vi "Core Actor - Init User Events.vi"(8 "error in (no error)":errorcluster, 11 "Parent_Class in":refnum<class "Message_Distributor_Class.lvclass">) -> (0 "error out":errorcluster, 3 "Parent_Class out":refnum<class "Message_Distributor_Class.lvclass">)   [LabVIEW 2023, in "Actor_Message_Distributor.lvlib" / "Message_Distributor_Class.lvclass"]
uses:
  Message_Distributor_Class.lvclass
  Usr Ev/Distributor - Ctrl - Action.ctl
  Message_Distributor_Class.lvclass/Message_Distributor_Class.ctl
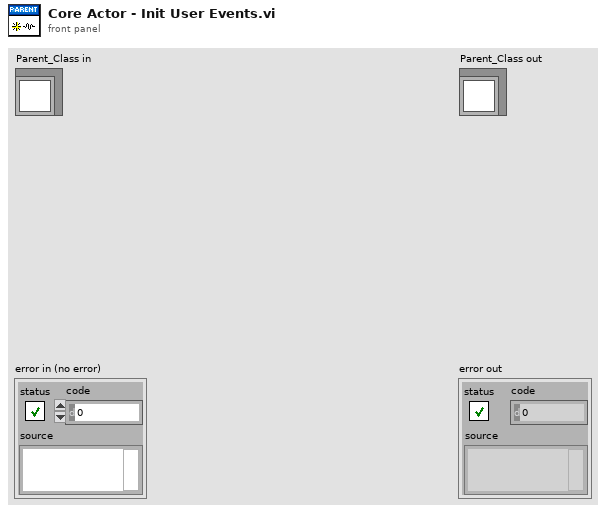
[diagram p1: front panel]
types:
  T1 = typedef "Actor_Message_Distributor.lvlib/Message_Distributor_Class.lvclass/Distributor - Ctrl - Action.ctl" = enum16{"Reg Ev", "Get Refs", "Close Ev", "Populate Enum with Events"}
  T2 = typedef "Actor_Message_Distributor.lvlib/Message_Distributor_Class.lvclass/Distributor - Ctrl - Usr Ev Ref.ctl" = cluster{"SEND MESSAGE Ev":cluster{"Data":refnum<user-event>}, "STOP_ACTOR Ev":cluster{"Data":refnum<user-event>}, "INIT_ACTOR Ev":cluster{"Data":refnum<user-event>}, "START Ev":cluster{"Data":refnum<user-event>}, "STOP Ev":cluster{"Data":refnum<user-event>}, "GET Ev":cluster{"Data":refnum<user-event>}, "SET Ev":cluster{"Data":refnum<user-event>}, "ERROR_HANDLER Ev":cluster{"Data":refnum<user-event>}, "RESET Ev":cluster{"Data":refnum<user-event>}, "DISPATCH MESSAGE 2 CHILDS Ev":cluster{"Data":refnum<user-event>}, "ECU RESET Ev":cluster{"Data":refnum<user-event>}, "T4 Ev":cluster{"Data":refnum<user-event>}}
  T3 = typedef "Actor_Message_Distributor.lvlib/Message_Distributor_Class.lvclass/Distributor - Ctrl - Usr Ev Reg - Refs.ctl" = cluster{"ERR1":refnum<event-registration>, "ERR2":refnum<event-registration>, "ERR3":refnum<event-registration>, "ERR4":refnum<event-registration>, "ERR5":refnum<event-registration>}
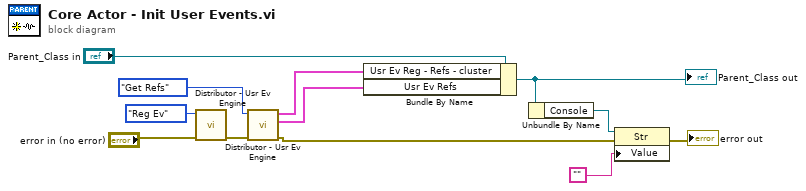
[diagram p0: block diagram]
diagram:
  n1 = call "Distributor - Usr Ev Engine.vi"("error in (no error)"="error in (no error)", "Action"=Distributor_-_Ctrl_-_Action."Reg Ev") -> ("error out"=w10:errorcluster)  [unwired: 6 in, 3 out]
  n2 = call "Distributor - Usr Ev Engine.vi"("error in (no error)"=w10, "Action"=Distributor_-_Ctrl_-_Action."Get Refs") -> ("error out"=w2:errorcluster, "Usr Ev Refs"=w6:T2, "Usr Ev Reg - Refs - cluster"=w7:T3)  [unwired: 6 in, 1 out]
  n3 = Bundle By Name(cluster="Parent_Class in", "Usr Ev Reg - Refs - cluster"=w7, "Usr Ev Refs"=w6) -> (w5:refnum<class "Message_Distributor_Class.lvclass">)
  "Parent_Class out" <- w5
  n4 = Unbundle By Name(w5) -> ("Console"=w3:refnum<vi>)
  n5 = property class="Str"(reference=w3, error in=w2, "Value"="") -> (error out=→"error out":errorcluster)  [unwired: 1 out]
